vi "ITBRead.vi"(0 "error in":errorcluster, 2 "Component":T2 items=["left_itb", "right_itb", "torso_left_itb", "torso_right_itb"], 3 "node":string) -> (1 "error out":errorcluster, 4 "ITB":T1)   [LabVIEW 2013]
doc: "This VI gets the status of the Navigator Buttons"
uses:
  ROS/Code/SubVIs/BaxterButtons.ctl
panel:
  in  "index":i32=8
  out "Reply":string
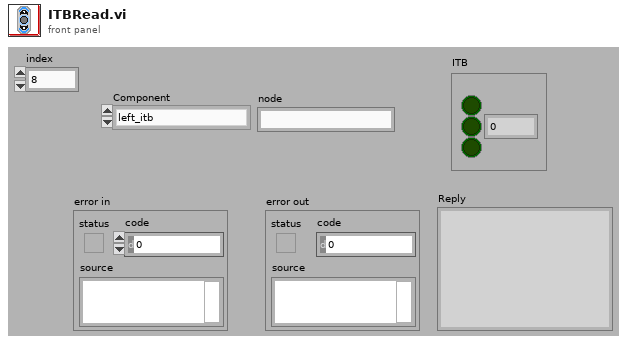
[diagram p1: front panel]
types:
  T1 = cluster{"Cancel":bool, "OK":bool, "Show":bool, "Wheel":u8}
  T2 = typedef "BaxterButtons.ctl" = u16
  T3 = typedef "_ROSControl.ctl" = cluster{"topic port":u16, "Node":string, "topic":string, "type":string, "node port":u32, "error ":errorcluster, "Direction":T4, "APIs":string[]}
  T4 = typedef "_ROSDirection.ctl" = enum16{"Node", "Publisher", "Subscriber", "Service Client"}
  T5 = cluster{"OK":bool, "Cancel":bool, "Show":bool, "Wheel":u8}
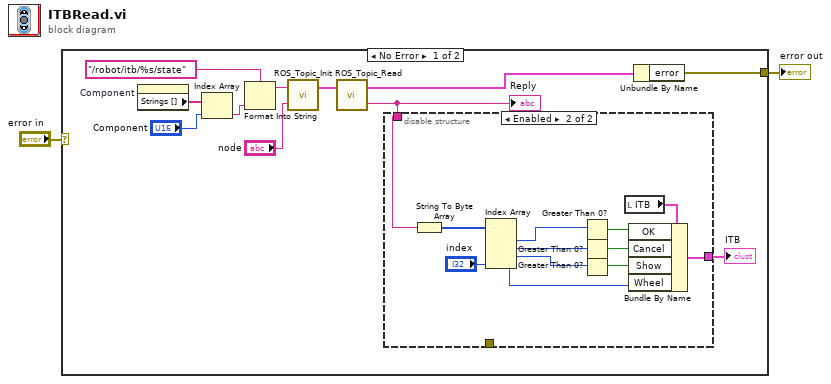
[diagram p0: block diagram]
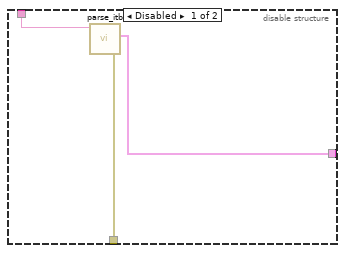
[diagram p2: hidden frame]
diagram:
  n1 = case shown="No Error" "error in" {
    selector: "error in" -> [_ w29]
    tunnel: [w13 w29] -> w2
    frame No Error {
      n2 = property on="Component" class="Ring (strict)"() -> ("Strings []"=w9:string[])  [unwired: 2 in, 2 out]
      n3 = Index Array(array=w9, index="Component") -> (element=w6:string)
      n4 = Format Into String(format string="/robot/itb/%s/state" ("topic"), w6) -> (resulting string=w5:string)  [unwired: 2 in, 1 out]
      n5 = call "ROS_Topic_Init.vi"("node"="node", "topic"=w5) -> ("ROS out"=w11:T3)  [unwired: 1 in]
      n6 = call "ROS_Topic_Read.vi"("ROS in"=w11) -> ("Reply"=w4:string, "ROS out"=w10:T3)  [unwired: 1 in]
      "Reply" <- w4
      n7 = disable-structure shown="Enabled" {
        disable-tunnel: w4 -> [w16 w26]
        disable-tunnel: [w15 w27] -> w3
        disable-tunnel: [w14 _] -> _
        frame Disabled {
          n8 = call "parse_itb.vi"("msg in"=w16) -> ("error out"=w14:errorcluster, "Navigator Inputs"=w15:T5)  [unwired: 4 in, 1 out]
        }
        frame Enabled {
          n9 = String To Byte Array(string=w26) -> (unsigned byte array=w25:u8[])
          n10 = Index Array(array=w25, index #4="index") -> (element #1=w21:u8, element #2=w20:u8, element #3=w19:u8, element #4=w18:u8)  [unwired: 3 in]
          n11 = Greater Than 0?(x=w21) -> (x > 0?=w24:bool)
          n12 = Greater Than 0?(x=w20) -> (x > 0?=w23:bool)
          n13 = Greater Than 0?(x=w19) -> (x > 0?=w22:bool)
          n14 = local read "ITB"() -> (w28:T1)
          n15 = Bundle By Name(cluster=w28, "OK"=w24, "Cancel"=w23, "Show"=w22, "Wheel"=w18) -> (w27:T1)
        }
      }
      "ITB" <- w3
      n16 = Unbundle By Name(w10) -> ("error"=w13:errorcluster)
    }
    frame Error {
    }
  }
  "error out" <- w2
